vi "EnqueData.vi"(8 "error in (no error)":errorcluster, 9 "EnqueForClusDisp":bool, 10 "EnqueForChanDisp (T)":bool=TRUE, 11 "DataReceiver in":refnum<class "DataReceiver.lvclass">) -> (0 "error out":errorcluster, 3 "DataReceiver out":refnum<class "DataReceiver.lvclass">)   [LabVIEW 2010, in "DataReceiver.lvclass"]
uses:
  DataReceiver.lvclass
  DataReceiver.lvclass/DataReceiver.ctl
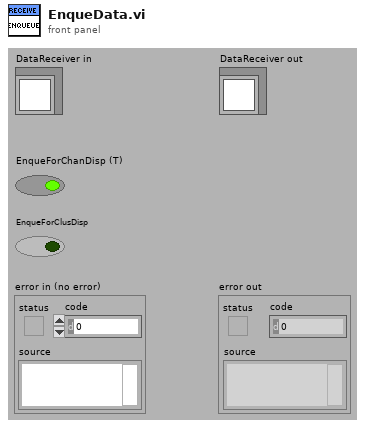
[diagram p1: front panel]
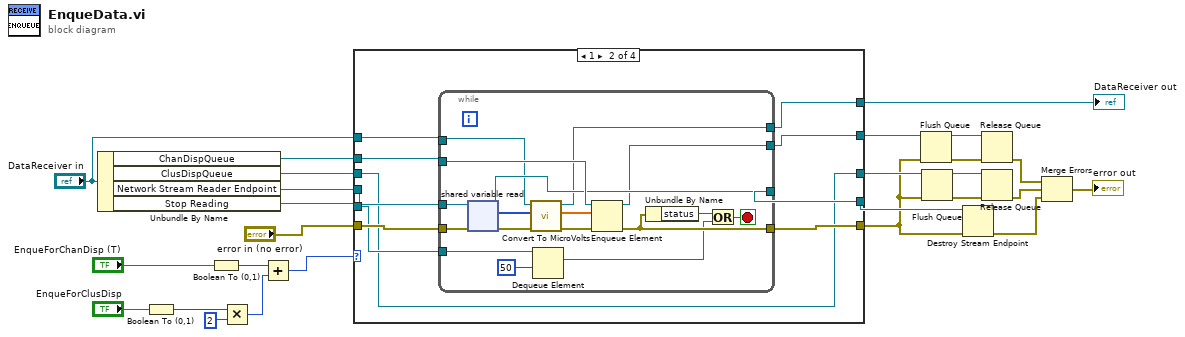
[diagram p0: block diagram]
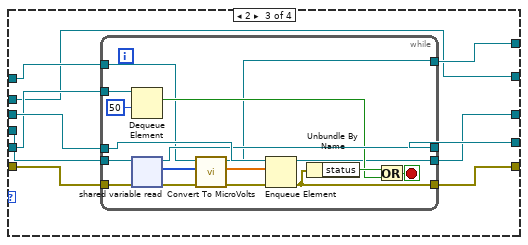
[diagram p3: hidden frame]
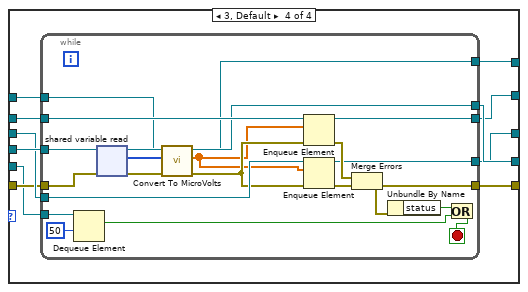
[diagram p4: hidden frame]
diagram:
  n1 = Unbundle By Name("DataReceiver in") -> ("ChanDispQueue"=w24:refnum<queue>, "ClusDispQueue"=w23:refnum<queue>, "Network Stream Reader Endpoint"=w15:refnum<k21>, "Stop Reading"=w13:refnum<queue>)
  n2 = Boolean To (0,1)(Boolean="EnqueForClusDisp") -> (0, 1=w22:i16)
  n3 = Boolean To (0,1)(Boolean="EnqueForChanDisp (T)") -> (0, 1=w20:i16)
  n4 = Multiply(x=w22, y=i16 2) -> (x*y=w19:i16)
  n5 = Add(x=w20, y=w19) -> (x+y=w18:i16)
  n6 = case shown="1" w18 {
    tunnel: w15 -> [w30 w40 w67 w96]
    tunnel: w24 -> [w28 w41 w60 w95]
    tunnel: w23 -> [w27 w33 w68 w94]
    tunnel: "error in (no error)" -> [w31 w39 w66 w93]
    tunnel: [w31 w38 w65 w92] -> w6
    tunnel: [w30 w37 w64 w91] -> w17
    tunnel: "DataReceiver in" -> [w29 w35 w62 w89]
    tunnel: w13 -> [_ w36 w63 w90]
    tunnel: [w29 w34 w61 w88] -> w12
    tunnel: [w28 w32 w60 w86] -> w9
    tunnel: [w27 w33 w59 w87] -> w8
    frame 0 {
    }
    frame 1 {
      n7 = while {
        tunnel: w40 -> [w58]
        tunnel: w41 -> [w57]
        tunnel: w39 -> [w56]
        tunnel: [w55] -> w38
        tunnel: [w54] -> w37
        tunnel: w36 -> [w51]
        tunnel: w35 -> [w47]
        tunnel: [w46] -> w34
        tunnel: [w43] -> w32
        stop <- w52 stop-if-true
        n8 = shared-variable-read(w58, w56) -> (w54:refnum<k21>, w49:errorcluster, w45:i32[])  [unwired: 1 in, 1 out]
        n9 = call-dynamic "Convert To MicroVolts.vi"("error in (no error)"=w49, "Raw Data"=w45, "DataReceiver in"=w47) -> ("error out"=w48:errorcluster, "microVolts"=w44:dbl[], "DataReceiver out"=w46:refnum<class "DataReceiver.lvclass">)  [unwired: 6 in]
        n10 = Dequeue Element(queue=w51, timeout in ms (-1)=50) -> (element=w50:bool)  [unwired: 1 in, 3 out]
        n11 = Enqueue Element(queue=w57, element=w44, error in (no error)=w48) -> (queue out=w43:refnum<queue>, error out=w55:errorcluster)  [unwired: 1 in, 1 out]
        n12 = Unbundle By Name(w55) -> ("status"=w53:bool)
        n13 = Or(x=w53, y=w50) -> (x .or. y?=w52:bool)
      }
    }
    frame 2 {
      n14 = while {
        tunnel: w67 -> [w85]
        tunnel: w68 -> [w84]
        tunnel: w66 -> [w83]
        tunnel: [w82] -> w65
        tunnel: [w81] -> w64
        tunnel: w63 -> [w80]
        tunnel: w62 -> [w73]
        tunnel: [w72] -> w61
        tunnel: [w70] -> w59
        stop <- w79 stop-if-true
        n15 = Dequeue Element(queue=w80, timeout in ms (-1)=50) -> (element=w77:bool)  [unwired: 1 in, 3 out]
        n16 = shared-variable-read(w85, w83) -> (w81:refnum<k21>, w76:errorcluster, w74:i32[])  [unwired: 1 in, 1 out]
        n17 = call-dynamic "Convert To MicroVolts.vi"("error in (no error)"=w76, "Raw Data"=w74, "DataReceiver in"=w73) -> ("error out"=w75:errorcluster, "microVolts"=w71:dbl[], "DataReceiver out"=w72:refnum<class "DataReceiver.lvclass">)  [unwired: 6 in]
        n18 = Enqueue Element(queue=w84, element=w71, error in (no error)=w75) -> (queue out=w70:refnum<queue>, error out=w82:errorcluster)  [unwired: 1 in, 1 out]
        n19 = Unbundle By Name(w82) -> ("status"=w78:bool)
        n20 = Or(x=w78, y=w77) -> (x .or. y?=w79:bool)
      }
    }
    frame 3, Default {
      n21 = while {
        tunnel: w96 -> [w117]
        tunnel: w95 -> [w116]
        tunnel: w94 -> [w115]
        tunnel: w93 -> [w114]
        tunnel: [w111] -> w92
        tunnel: [w110] -> w91
        tunnel: w90 -> [w108]
        tunnel: w89 -> [w103]
        tunnel: [w102] -> w88
        tunnel: [w99] -> w86
        tunnel: [w98] -> w87
        stop <- w106 stop-if-true
        n22 = Dequeue Element(queue=w108, timeout in ms (-1)=50) -> (element=w109:bool)  [unwired: 1 in, 3 out]
        n23 = shared-variable-read(w117, w114) -> (w110:refnum<k21>, w105:errorcluster, w101:i32[])  [unwired: 1 in, 1 out]
        n24 = call-dynamic "Convert To MicroVolts.vi"("error in (no error)"=w105, "Raw Data"=w101, "DataReceiver in"=w103) -> ("error out"=w104:errorcluster, "microVolts"=w100:dbl[], "DataReceiver out"=w102:refnum<class "DataReceiver.lvclass">)  [unwired: 6 in]
        n25 = Enqueue Element(queue=w116, element=w100, error in (no error)=w104) -> (queue out=w99:refnum<queue>, error out=w113:errorcluster)  [unwired: 1 in, 1 out]
        n26 = Enqueue Element(queue=w115, element=w100, error in (no error)=w104) -> (queue out=w98:refnum<queue>, error out=w112:errorcluster)  [unwired: 1 in, 1 out]
        n27 = Merge Errors(w113, w112) -> (w111:errorcluster)
        n28 = Unbundle By Name(w111) -> ("status"=w107:bool)
        n29 = Or(x=w107, y=w109) -> (x .or. y?=w106:bool)
      }
    }
  }
  "DataReceiver out" <- w12
  n30 = Flush Queue(queue=w9, error in (no error)=w6) -> (queue out=w7:refnum<queue>, error out=w5:errorcluster)  [unwired: 1 out]
  n31 = Flush Queue(queue=w8, error in (no error)=w6) -> (queue out=w11:refnum<queue>, error out=w10:errorcluster)  [unwired: 1 out]
  n32 = Destroy Stream Endpoint(8:w6, 11:w17) -> (0:w2:errorcluster)
  n33 = Release Queue(queue=w7, error in (no error)=w5) -> (error out=w3:errorcluster)  [unwired: 1 in, 2 out]
  n34 = Release Queue(queue=w11, error in (no error)=w10) -> (error out=w4:errorcluster)  [unwired: 1 in, 2 out]
  n35 = Merge Errors(w3, w4, w2) -> (→"error out":errorcluster)
